vi "Configure AC Real Current Limit.vi"(6 "Mode":u16(ring) items=["AC"], 7 "error in (no error)":errorcluster, 8 "Real Current Limit [A]":dbl=1e-05 min=1e-05 max=0.005 step=1e-05 format="%.3p", 9 "Step":T1=1 min=1 max=99 step=1, 10 "VISA resource name":refnum<visa-resource-name>) -> (0 "error out":errorcluster, 3 "VISA resource name out":refnum<visa-resource-name>)   [LabVIEW 2025]
uses:
  <instrlib>/Chrome 19025/Public/Utility/Type Def/steps--numeric.ctl
panel:
  # "Configure Real Current Limit"
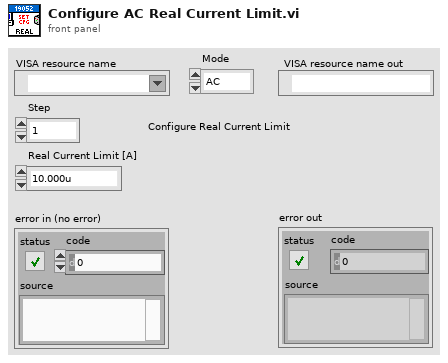
[diagram p1: front panel]
types:
  T1 = typedef "Chrome 19025.lvlib/steps--numeric.ctl" = u8
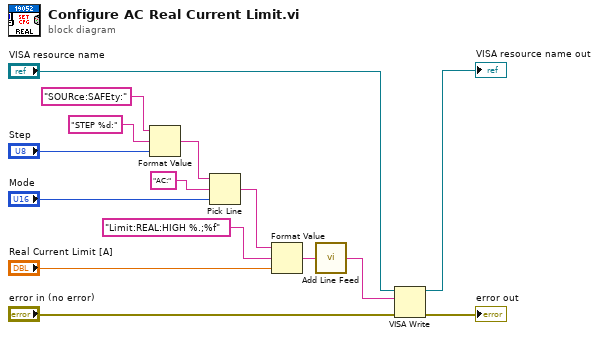
[diagram p0: block diagram]
diagram:
  n1 = Format Value(string ("")="SOURce:SAFEty:", format string="STEP %d:", value (0)="Step") -> (output string=w10:string)
  n2 = Pick Line(string ("")=w10, multi-line string="AC:", line index="Mode") -> (output string=w7:string)
  n3 = Format Value(string ("")=w7, format string="Limit:REAL:HIGH %.;%f", value (0)="Real Current Limit [A]") -> (output string=w6:string)
  n4 = call <instrlib>:"Add Line Feed.vi"("Command string"=w6) -> ("Concatenated string"=w5:string)  [unwired: 4 in]
  n5 = VISA Write(VISA resource name="VISA resource name", write buffer=w5, error in (no error)="error in (no error)") -> (VISA resource name out=→"VISA resource name out":refnum<visa-resource-name>, error out=→"error out":errorcluster)  [unwired: 1 out]
